vi "JEOL_SEM.vi"() -> ()   [LabVIEW 2016]
uses:
  cluster_fontsettings.ctl
  cluster_colorsettings.ctl
  cluster_spacing.ctl
  cluster_background.ctl
panel:
  out "picture":picture
  in  "save all images":bool
  in  "End Program":bool
  out "Resolution [px]":i16[](array[numeric])=[2560, 1920] caption="Picture resolution (X*Y = width x height) [pixel]"
  in  "Spacing":T1={"Background"={"use picture width"=FALSE, "Settings"={"add box below image"=FALSE, "extra width background"=30, "extra height background"=30, "x [px]"=50.0, "y [px]"=50.0}}, "Scalebar"={"height of bar [px]"=50.0, "width scaling factor"=1.0, "Precision"=0}}
  in  "Color settings":T3={"Background color"=0, "Information color"=16777215}
  in  "Font settings":T4={"Font"=0, "Font size [px]"=60, "Bold"=FALSE} {"Font" items=["Arial", "Arial Italic", "Arial Bold", "Arial Bold Italic", "Batang & BatangChe & Gungsuh & GungsuhChe", "Courier New", "Courier New Italic", "Courier New Bold", "Courier New Bold Italic", "DaunPenh", "DokChampa", "Estrangelo Edessa", "Euphemia", "Gautami", "Gautami Bold", "Vani", "Vani Bold", "Gulim & GulimChe & Dotum & DotumChe", "Impact", "Iskoola Pota", "Iskoola Pota Bold", "Kalinga", "Kalinga Bold", "Kartika", "Kartika Bold", "Khmer UI", "Khmer UI Bold", "Lao UI", "Lao UI Bold", "Latha", "Latha Bold", "Lucida Console", "Malgun Gothic", "Malgun Gothic Bold", "Mangal", "Mangal Bold", "Meiryo & Meiryo Italic & Meiryo UI & Meiryo UI Italic", "Meiryo Bold & Meiryo Bold Italic & Meiryo UI Bold & Meiryo UI Bold Italic", "Microsoft Himalaya", "Microsoft JhengHei", "Microsoft JhengHei Bold", "Microsoft YaHei", "Microsoft YaHei Bold", "MingLiU & PMingLiU & MingLiU_HKSCS", "MingLiU-ExtB & PMingLiU-ExtB & MingLiU_HKSCS-ExtB", "Mongolian Baiti", "MS Gothic & MS PGothic & MS UI Gothic", "MS Mincho & MS PMincho", "MV Boli", "Microsoft New Tai Lue", "Microsoft New Tai Lue Bold", "Nyala", "Microsoft PhagsPa", "Microsoft PhagsPa Bold", "Plantagenet Cherokee", "Raavi", "Raavi Bold", "Segoe Script", "Segoe Script Bold", "Segoe UI", "Segoe UI Bold", "Segoe UI Italic", "Segoe UI Bold Italic", "Segoe UI Semibold", "Segoe UI Light", "Segoe UI Symbol", "Shruti", "Shruti Bold", "SimSun & NSimSun", "SimSun-ExtB", "Sylfaen", "Microsoft Tai Le", "Microsoft Tai Le Bold", "Times New Roman", "Times New Roman Italic", "Times New Roman Bold", "Times New Roman Bold Italic", "Tunga", "Tunga Bold", "Vrinda", "Vrinda Bold", "Shonar Bangla", "Shonar Bangla Bold", "Microsoft Yi Baiti", "Tahoma", "Tahoma Bold", "Microsoft Sans Serif", "Angsana New", "Angsana New Italic", "Angsana New Bold", "Angsana New Bold Italic", "Aparajita", "Aparajita Bold", "Aparajita Bold Italic(TrueType)", "Aparajita Italic", "Cordia New", "Cordia New Italic", "Cordia New Bold", "Cordia New Bold Italic", "Ebrima", "Ebrima Bold", "Gisha", "Gisha Bold", "Kokila", "Kokila Bold", "Kokila Bold Italic(TrueType)", "Kokila Italic", "MoolBoran", "Symbol", "Utsaah", "Utsaah Bold", "Utsaah Bold Italic(TrueType)", "Utsaah Italic", "Vijaya", "Vijaya Bold", "Wingdings", "Modern", "Roman", "Script", "Andalus", "Arabic Typesetting", "Simplified Arabic", "Simplified Arabic Bold", "Simplified Arabic Fixed", "Sakkal Majalla", "Sakkal Majalla Bold", "Traditional Arabic", "Traditional Arabic Bold", "Aharoni Bold", "David", "David Bold", "FrankRuehl", "Levenim MT", "Levenim MT Bold", "Miriam", "Miriam Fixed", "Narkisim", "Rod", "FangSong", "SimHei", "KaiTi", "AngsanaUPC", "AngsanaUPC Italic", "AngsanaUPC Bold", "AngsanaUPC Bold Italic", "Browallia New", "Browallia New Italic", "Browallia New Bold", "Browallia New Bold Italic", "BrowalliaUPC", "BrowalliaUPC Italic", "BrowalliaUPC Bold", "BrowalliaUPC Bold Italic", "CordiaUPC", "CordiaUPC Bold", "CordiaUPC Bold Italic", "CordiaUPC Italic", "DilleniaUPC", "DilleniaUPC Italic", "DilleniaUPC Bold", "DilleniaUPC Bold Italic", "EucrosiaUPC", "EucrosiaUPC Italic", "EucrosiaUPC Bold", "EucrosiaUPC Bold Italic", "FreesiaUPC", "FreesiaUPC Italic", "FreesiaUPC Bold", "FreesiaUPC Bold Italic", "IrisUPC", "IrisUPC Italic", "IrisUPC Bold", "IrisUPC Bold Italic", "JasmineUPC", "JasmineUPC Italic", "JasmineUPC Bold", "JasmineUPC Bold Italic", "KodchiangUPC", "KodchiangUPC Italic", "KodchiangUPC Bold", "KodchiangUPC Bold Italic", "LilyUPC", "LilyUPC Italic", "LilyUPC Bold", "LilyUPC Bold Italic", "DFKai-SB", "Lucida Sans Unicode", "Arial Black", "Calibri", "Calibri Italic", "Calibri Bold", "Calibri Bold Italic", "Cambria & Cambria Math", "Cambria Italic", "Cambria Bold", "Cambria Bold Italic", "Candara", "Candara Italic", "Candara Bold", "Candara Bold Italic", "Comic Sans MS", "Comic Sans MS Bold", "Consolas", "Consolas Italic", "Consolas Bold", "Consolas Bold Italic", "Constantia", "Constantia Italic", "Constantia Bold", "Constantia Bold Italic", "Corbel", "Corbel Italic", "Corbel Bold", "Corbel Bold Italic", "Franklin Gothic Medium", "Franklin Gothic Medium Italic", "Gabriola", "Georgia", "Georgia Italic", "Georgia Bold", "Georgia Bold Italic", "Palatino Linotype", "Palatino Linotype Italic", "Palatino Linotype Bold", "Palatino Linotype Bold Italic", "Segoe Print", "Segoe Print Bold", "Trebuchet MS", "Trebuchet MS Italic", "Trebuchet MS Bold", "Trebuchet MS Bold Italic", "Verdana", "Verdana Italic", "Verdana Bold", "Verdana Bold Italic", "Webdings", "Courier 10,12,15", "MS Serif 8,10,12,14,18,24", "MS Sans Serif 8,10,12,14,18,24", "Small Fonts", "Small Fonts", "Arial Narrow", "Book Antiqua", "Bookman Old Style", "Century Gothic", "Garamond", "Monotype Corsiva", "Book Antiqua Bold", "Book Antiqua Bold Italic", "Book Antiqua Italic", "Arial Narrow Bold", "Arial Narrow Bold Italic", "Arial Narrow Italic", "Bookman Old Style Bold", "Bookman Old Style Bold Italic", "Bookman Old Style Italic", "Garamond Bold", "Garamond Italic", "Century Gothic Bold", "Century Gothic Bold Italic", "Century Gothic Italic", "DIN-Bold", "DIN-Regular", "DIN-Black", "BEYBNQ+InfoDispRegular-Roman", "motorhead Standard", "FENCES.TTF", "MTEXTRA.TTF", "Origin", "Roboto Condensed Light Italic", "Roboto Condensed Regular", "Roboto Condensed Bold Italic", "Roboto Condensed Italic", "Roboto Condensed Light", "LMSans10-Regular", "LMSans10-BoldOblique", "LMSans10-Oblique", "LMSans10-Bold", "LMSansDemiCond10-Oblique", "Roboto Condensed Bold", "FA123ALG", "FA123GRF", "Agency FB Fett", "Agency FB", "Algerian", "Arial Rounded MT Bold", "Baskerville Old Face", "Bauhaus 93", "Bell MT", "Bell MT Fett", "Bell MT Kursiv", "Bernard MT Condensed", "Bodoni MT Fett", "Bodoni MT Fett Kursiv", "Bodoni MT Black Kursiv", "Bodoni MT Black", "Bodoni MT Condensed Fett", "Bodoni MT Condensed Fett Kursiv", "Bodoni MT Condensed Kursiv", "Bodoni MT Condensed", "Bodoni MT Kursiv", "Bodoni MT Poster Compressed", "Bodoni MT", "Bradley Hand ITC", "Britannic Bold", "Berlin Sans FB Fett", "Berlin Sans FB Demi Fett", "Berlin Sans FB", "Broadway", "Brush Script MT Kursiv", "Bookshelf Symbol 7", "Californian FB Fett", "Californian FB Kursiv", "Californian FB", "Calisto MT", "Calisto MT Fett", "Calisto MT Fett Kursiv", "Calisto MT Kursiv", "Castellar", "Century Schoolbook", "Centaur", "Chiller", "Colonna MT", "Cooper Black", "Copperplate Gothic Bold", "Copperplate Gothic Light", "Curlz MT", "Elephant", "Elephant Kursiv", "Engravers MT", "Eras Bold ITC", "Eras Demi ITC", "Eras Light ITC", "Eras Medium ITC", "Felix Titling", "Forte", "Franklin Gothic Book", "Franklin Gothic Book Kursiv", "Franklin Gothic Demi", "Franklin Gothic Demi Cond", "Franklin Gothic Demi Kursiv", "Franklin Gothic Heavy", "Franklin Gothic Heavy Kursiv", "Franklin Gothic Medium Cond", "Freestyle Script", "French Script MT", "Footlight MT Light", "Gigi", "Gill Sans MT", "Gill Sans MT Fett", "Gill Sans MT Fett Kursiv", "Gill Sans MT Condensed", "Gill Sans MT Kursiv", "Gill Sans Ultra Bold Condensed", "Gill Sans Ultra Bold", "Gloucester MT Extra Condensed", "Gill Sans MT Ext Condensed Bold", "Goudy Old Style", "Goudy Old Style Fett", "Goudy Old Style Kursiv", "Goudy Stout", "Harlow Solid Italic", "Harrington", "Haettenschweiler", "High Tower Text", "High Tower Text Kursiv", "Imprint MT Shadow", "Informal Roman", "Blackadder ITC", "Edwardian Script ITC", "Kristen ITC", "Jokerman", "Juice ITC", "Kunstler Script", "Wide Latin", "Lucida Bright", "Lucida Bright Demibold", "Lucida Bright Demibold Italic", "Lucida Bright Italic", "Lucida Calligraphy Italic", "Lucida Fax", "Lucida Fax Halbfett", "Lucida Fax Halbfett Kursiv", "Lucida Fax Kursiv", "Lucida Handwriting Kursiv", "Lucida Sans", "Lucida Sans Halbfett", "Lucida Sans Halbfett Kursiv", "Lucida Sans Kursiv", "Lucida Sans Typewriter", "Lucida Sans Typewriter Fett", "Lucida Sans Typewriter Fett Schräg", "Lucida Sans Typewriter Schräg", "Magneto Fett", "Maiandra GD", "Matura MT Script Capitals", "Mistral", "Modern No. 20", "Niagara Engraved", "Niagara Solid", "OCR A Extended", "Old English Text MT", "Onyx", "MS Outlook", "Palace Script MT", "Papyrus", "Parchment", "Perpetua", "Perpetua Fett", "Perpetua Fett Kursiv", "Perpetua Kursiv", "Perpetua Titling MT Fett", "Perpetua Titling MT Mager", "Playbill", "Poor Richard", "Pristina", "Rage Italic", "Ravie", "MS Reference Sans Serif", "MS Reference Specialty", "Rockwell Condensed", "Rockwell Condensed Fett", "Rockwell", "Rockwell Fett", "Rockwell Fett Kursiv", "Rockwell Extra Bold", "Rockwell Kursiv", "Century Schoolbook Fett", "Century Schoolbook Fett Kursiv", "Century Schoolbook Kursiv", "Script MT Bold", "Showcard Gothic", "Snap ITC", "Stencil", "Tw Cen MT Fett", "Tw Cen MT Fett Kursiv", "Tw Cen MT Condensed Fett", "Tw Cen MT Condensed Extra Bold", "Tw Cen MT Condensed", "Tw Cen MT", "Tw Cen MT Kursiv", "Tempus Sans ITC", "Viner Hand ITC", "Vivaldi Kursiv", "Vladimir Script", "Digital Readout Upright", "Eurotherm Message Center", "Eurotherm Starburst", "Eurotherm Series 2000", "FreeSerif Fett-Kursiv", "FreeSerif Fett", "FreeSerif Mittel", "FreeSans Kursiv", "FreeSans Fett-Kursiv", "FreeSans Fett", "FreeSans Mittel", "FreeMono Kursiv", "FreeMono Fett-Kursiv", "FreeMono Fett", "FreeMono Standard", "FreeSerif Kursiv", "TeamViewer12", "Arial Unicode MS", "Century", "Gadugi", "Leelawadee", "Microsoft JhengHei & Microsoft JhengHei UI", "Microsoft Uighur", "Microsoft YaHei & Microsoft YaHei UI", "Segoe UI Semilight", "Wingdings 2", "Wingdings 3", "Gadugi Bold", "Leelawadee Bold", "Microsoft JhengHei Bold & Microsoft JhengHei UI Bold", "Microsoft Uighur Bold", "Microsoft YaHei Bold & Microsoft YaHei UI Bold", "Nirmala UI Bold", "Calibri Light Italic", "Nirmala UI", "Calibri Light", "Leipzig Fraktur Normal", "MT Extra"]}
  in  "save image":bool
  in  "Preview":bool
  in  "load image":bool
  in  "Path to directory to convert all files (only save image will work, so make sure settings are ok!)":path
  in  "Path to single file (png or txt with metadata)":path
  # "x and y are the distance between the\nlower left corner of the image and the\nlower left corner of the box"
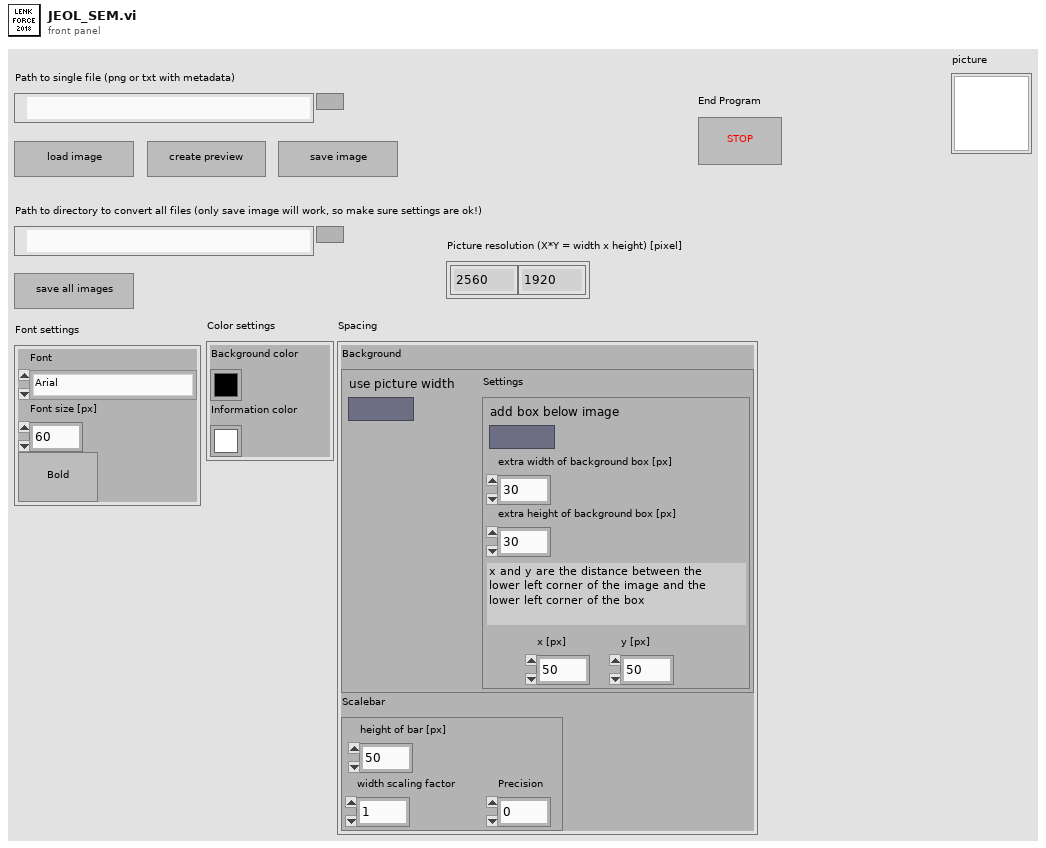
[diagram p1: front panel]
types:
  T1 = typedef "cluster_spacing.ctl" = cluster{"Background":T2, "Scalebar":cluster{"height of bar [px]":dbl, "width scaling factor":dbl, "Precision":i16}}
  T2 = typedef "cluster_background.ctl" = cluster{"use picture width":bool, "Settings":cluster{"add box below image":bool, "extra width background":i16, "extra height background":i16, "x [px]":dbl, "y [px]":dbl}}
  T3 = typedef "cluster_colorsettings.ctl" = cluster{"Background color":u32, "Information color":u32}
  T4 = typedef "cluster_fontsettings.ctl" = cluster{"Font":u16, "Font size [px]":i16, "Bold":bool}
  T5 = cluster{"Font Name:":string, "Size":i16, "Strikeout?":bool, "Italic?":bool, "Underline?":bool, "Outline?":bool, "Shadow?":bool, "Bold?":bool}
  T6 = typedef "cluster_metadata.ctl" = cluster{"FOV v":dbl, "FOV v unit":string, "FOV h":dbl, "FOV h unit":string, "Micron marker":dbl, "Micron marker unit":string, "Resolution h":i32, "Resolution v":i32, "Maginfication":i32}
  T7 = typedef "imagedata.ctl" = cluster{"image type":i32, "image depth":i32, "image":u8[], "mask":u8[], "colors":u32[], "Rectangle":cluster{"left":i16, "top":i16, "right":i16, "bottom":i16}}
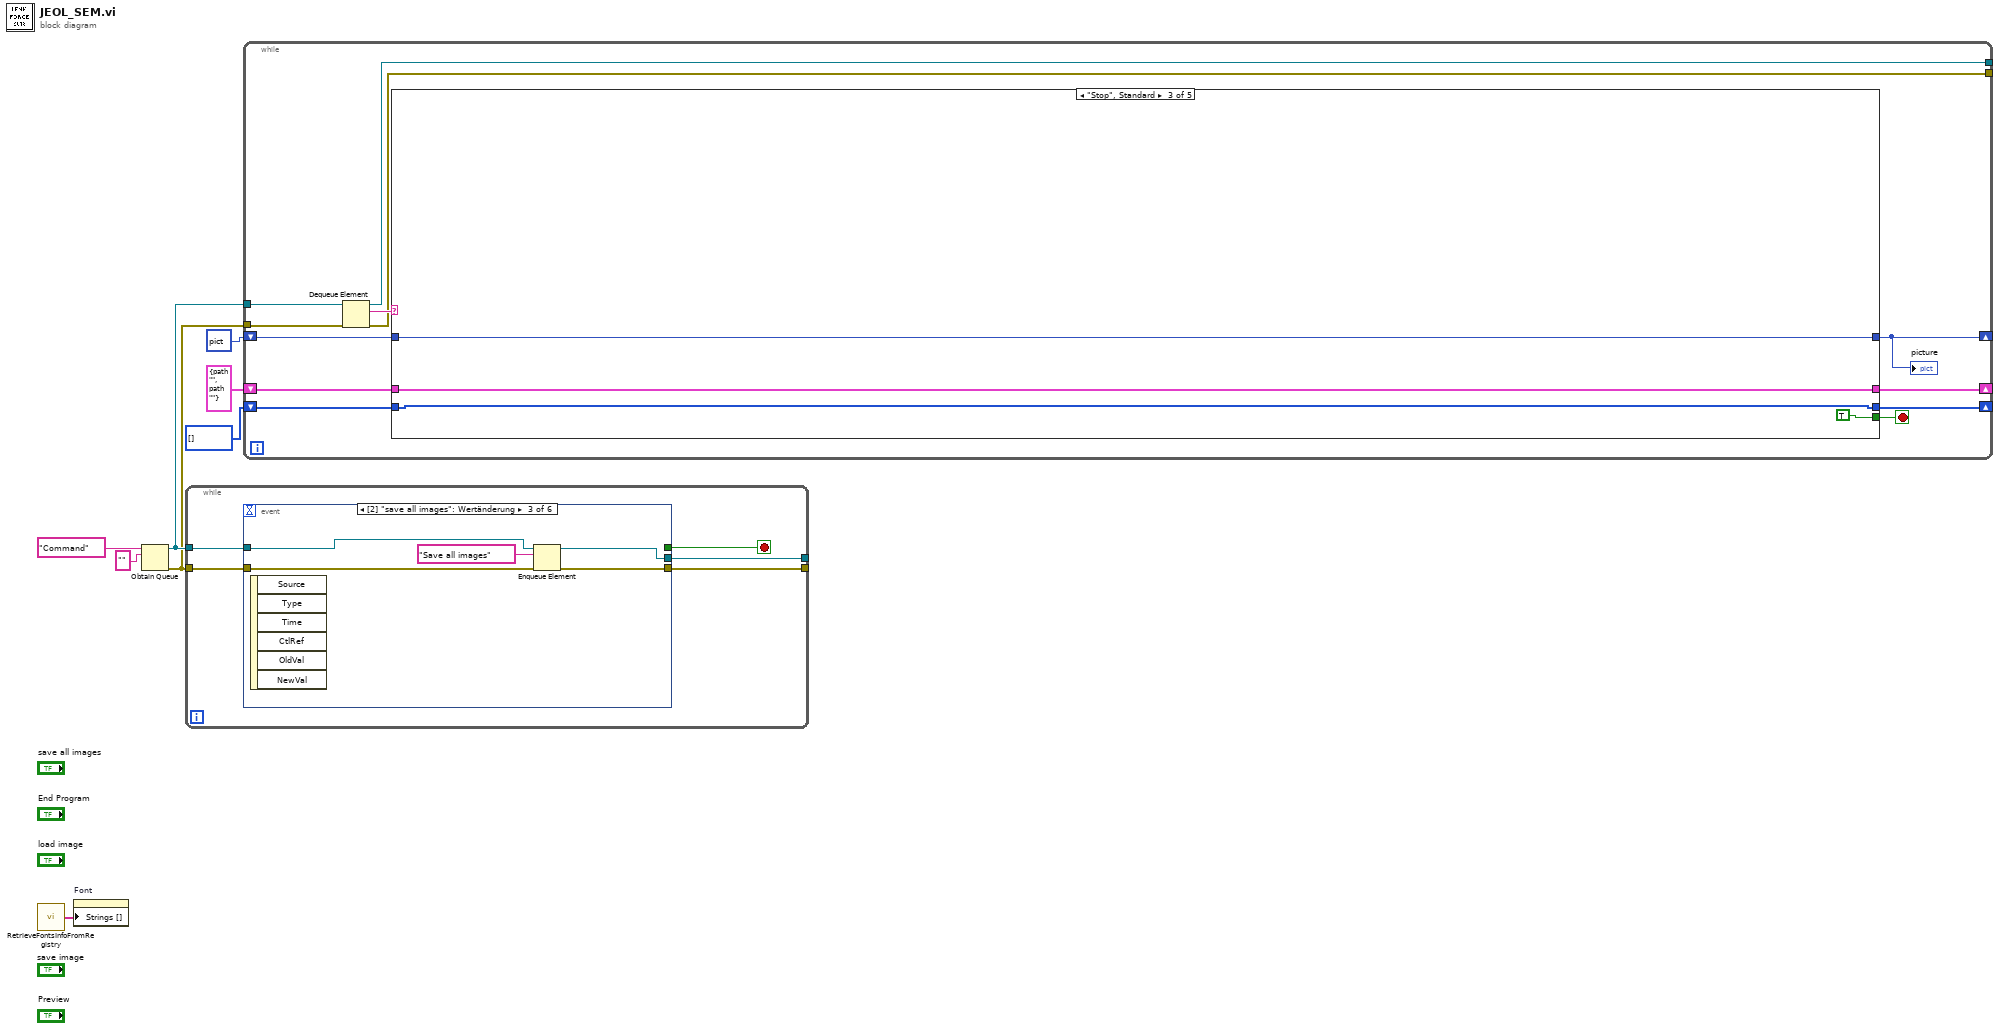
[diagram p0: block diagram]
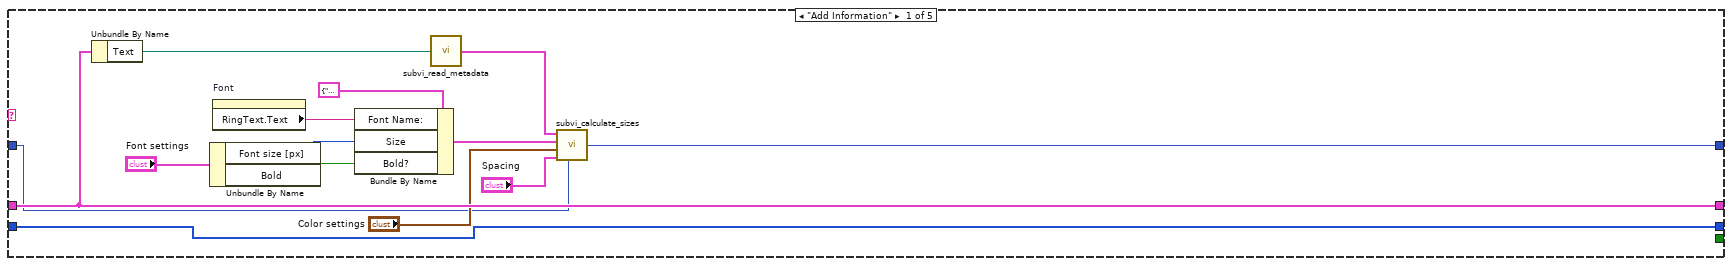
[diagram p2: hidden frame]
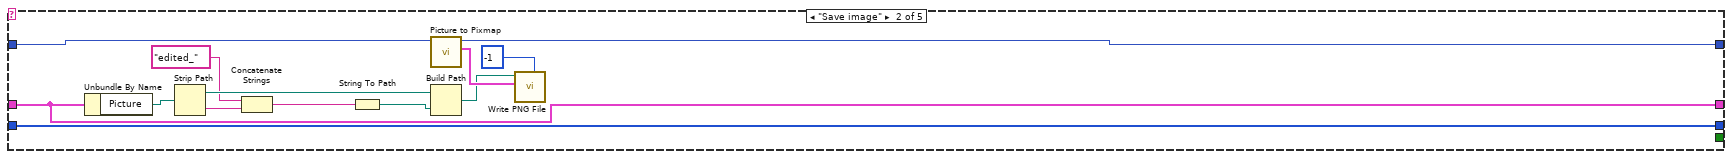
[diagram p3: hidden frame]
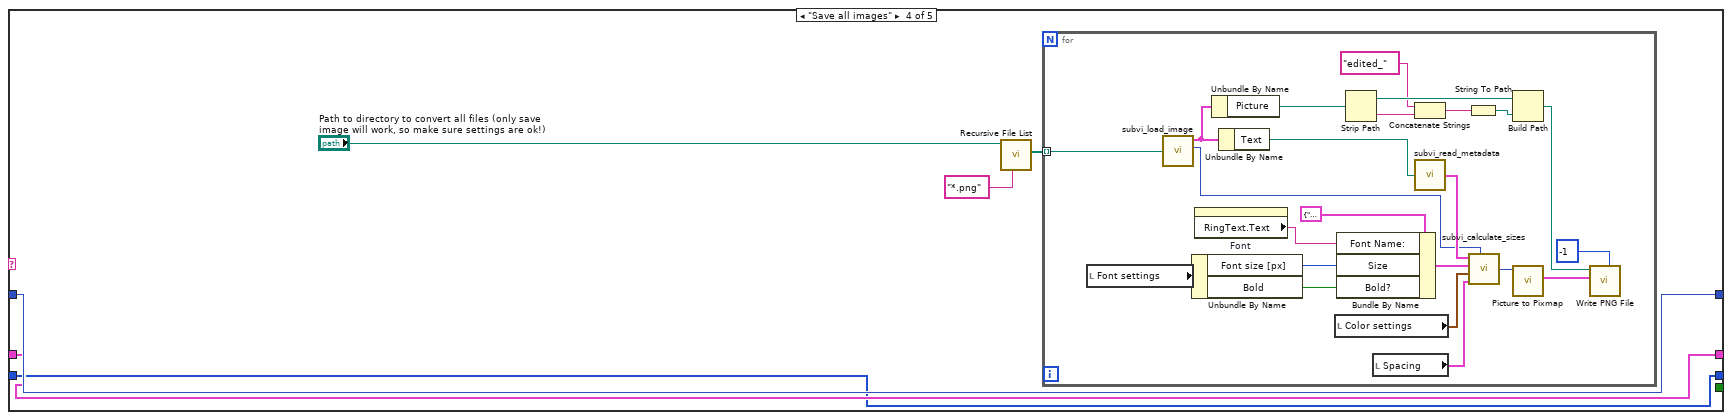
[diagram p4: hidden frame]
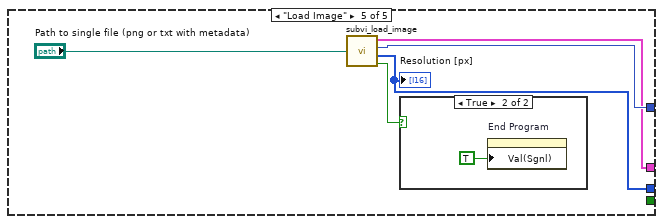
[diagram p5: hidden frame]
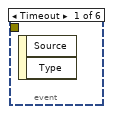
[diagram p7: hidden frame]
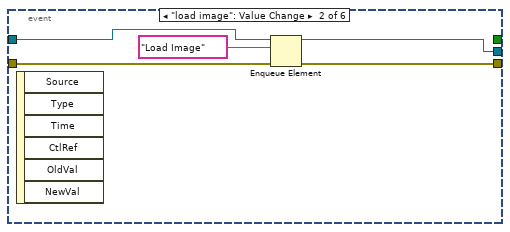
[diagram p8: hidden frame]
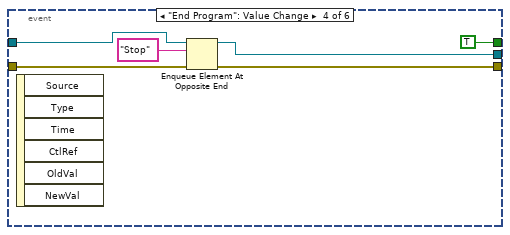
[diagram p9: hidden frame]
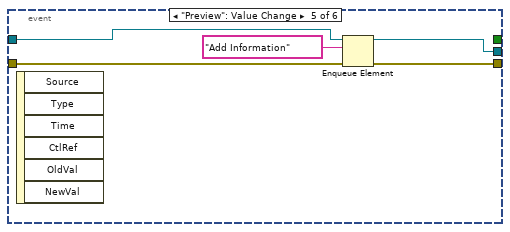
[diagram p10: hidden frame]
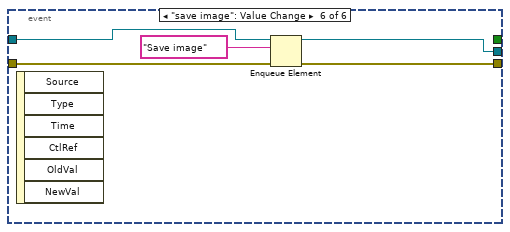
[diagram p11: hidden frame]
diagram:
  n1 = call "RetrieveFontsInfoFromRegistry.vi"() -> ("Fonts Installed"=w8:string[])
  n2 = property on="Font" class="Ring (strikt)"("Strings []"=w8) -> ()  [unwired: 2 in, 2 out]
  n3 = Obtain Queue(name (unnamed)="Command" ("Name (unbenannt)"), element data type="") -> (queue out=w6:refnum<queue>, error out=w4:errorcluster)  [unwired: 3 in, 1 out]
  n4 = while {
    tunnel: w6 -> [w13]
    tunnel: w4 -> [w12]
    tunnel: [w11] -> _
    tunnel: [w10] -> _
    stop <- w9 stop-if-true
    n5 = event shown="[2] \"save all images\": Wertänderung" {
      selector: _ -> [_ _ _ _ _ _]
      dyn-events: _ -> [_ _ _ _ _ _]
      timeout: _ -> [_ _ _ _ _ _]
      tunnel: w13 -> [_ w18 w22 w29 w34 w38]
      tunnel: w12 -> [_ w17 w21 w26 w33 w35]
      tunnel: [_ w15 w20 w28 w31 w37] -> w11
      tunnel: [_ w14 w19 w25 w32 w36] -> w10
      tunnel: [_ _ _ TRUE _ _] -> w9
      event Timeout {
        n6 = event-data() -> ()  [unwired: 1 in, 2 out]
      }
      event "load image": Value Change {
        n7 = event-data() -> ()  [unwired: 1 in, 6 out]
        n8 = Enqueue Element(queue=w18, element="Load Image" ("Element"), error in (no error)=w17) -> (queue out=w15:refnum<queue>, error out=w14:errorcluster)  [unwired: 1 in, 1 out]
      }
      event "save all images": Value Change {
        n9 = event-data() -> ()  [unwired: 1 in, 6 out]
        n10 = Enqueue Element(queue=w22, element="Save all images" ("Element"), error in (no error)=w21) -> (queue out=w20:refnum<queue>, error out=w19:errorcluster)  [unwired: 1 in, 1 out]
      }
      event "End Program": Value Change {
        n11 = event-data() -> ()  [unwired: 1 in, 6 out]
        n12 = Enqueue Element At Opposite End(queue=w29, element="Stop" ("Element"), error in (no error)=w26) -> (queue out=w28:refnum<queue>, error out=w25:errorcluster)  [unwired: 1 in, 1 out]
      }
      event "Preview": Value Change {
        n13 = event-data() -> ()  [unwired: 1 in, 6 out]
        n14 = Enqueue Element(queue=w34, element="Add Information" ("Element"), error in (no error)=w33) -> (queue out=w31:refnum<queue>, error out=w32:errorcluster)  [unwired: 1 in, 1 out]
      }
      event "save image": Value Change {
        n15 = event-data() -> ()  [unwired: 1 in, 6 out]
        n16 = Enqueue Element(queue=w38, element="Save image" ("Element"), error in (no error)=w35) -> (queue out=w37:refnum<queue>, error out=w36:errorcluster)  [unwired: 1 in, 1 out]
      }
    }
  }
  n17 = while {
    tunnel: w6 -> [w51]
    tunnel: w4 -> [w50]
    shift-right: [w48] -> _
    shift-left: picture data[5B] ("loaded picture") -> [w47]
    shift-right: [w46] -> _
    shift-left: i16[] [] ("Resolution [px]") -> [w45]
    shift-right: [w44] -> _
    shift-left: cluster{"Picture":path, "Text":path} {"Picture"=path "", "Text"=path ""} ("Paths to data") -> [w43]
    tunnel: [w41] -> _
    tunnel: [w40] -> _
    stop <- w42 stop-if-true
    n18 = Dequeue Element(queue=w51, error in (no error)=w50) -> (queue out=w41:refnum<queue>, element=w49:string, error out=w40:errorcluster)  [unwired: 1 in, 1 out]
    n19 = case shown="\"Stop\", Standard" w49 {
      tunnel: [w52 w75 w80 w85 w115] -> w48
      tunnel: w47 -> [w54 w76 w80 w85 _]
      tunnel: [w53 w69 w79 w83 w114] -> w46
      tunnel: w45 -> [w53 w69 w79 w83 _]
      tunnel: [w65 w70 w81 w84 w112] -> w44
      tunnel: w43 -> [w65 w70 w81 w84 _]
      tunnel: [_ _ TRUE _ _] -> w42
      frame "Add Information" {
        n20 = Unbundle By Name(w65) -> ("Text"=w64:path)
        n21 = Unbundle By Name("Font settings") -> ("Font size [px]"=w63:i16, "Bold"=w62:bool)
        n22 = property on="Font" class="Ring (strikt)"() -> ("RingText.Text"=w59:string)  [unwired: 2 in, 2 out]
        n23 = Bundle By Name(cluster=T5 {"Font Name:"="Arial", "Size"=12, "Strikeout?"=FALSE, "Italic?"=FALSE, "Underline?"=FALSE, "Outline?"=FALSE, "Shadow?"=FALSE, "Bold?"=FALSE} ("[user-specified font]"), "Font Name:"=w59, "Size"=w63, "Bold?"=w62) -> (w57:T5)
        n24 = call "subvi_read_metadata.vi"("Pfad"=w64) -> ("Metadata"=w58:T6)
        n25 = call "subvi_calculate_sizes.vi"("Metadata"=w58, "font settings"=w57, "Color settings"="Color settings", "Spacing"="Spacing", "loaded picture"=w54) -> ("modified pictures"=w52:picture)
      }
      frame "Save image" {
        n26 = Unbundle By Name(w70) -> ("Picture"=w74:path)
        n27 = Strip Path(path=w74) -> (stripped path=w73:path, name=w68:string)
        n28 = Concatenate Strings("edited_" ("String"), w68) -> (w66:string)
        n29 = String To Path(string=w66) -> (path=w72:path)
        n30 = call <vilib>:"Picture to Pixmap.vi"("picture"=w76) -> ("image data"=w77:T7, "new picture"=w75:picture)  [unwired: 9 in]
        n31 = Build Path(base path=w73, name or relative path=w72) -> (appended path=w71:path)
        n32 = call <vilib>:"Write PNG File.vi"("compression (default)"=-1, "image data"=w77, "path to PNG file"=w71) -> ()  [unwired: 7 in, 2 out]
      }
      frame "Stop", Default {
      }
      frame "Save all images" {
        n33 = call <vilib>:"Recursive File List.vi"("pattern"="*.png", "Folder Path"="Path to directory to convert all files (only save image will work, so make sure settings are ok!)") -> ("All Files in Dir"=w86:path[])  [unwired: 5 in, 4 out]
        n34 = for {
          tunnel: w86 -> [w111] mode=indexing
          n35 = local read "Font settings"() -> (w102:T4)
          n36 = call "subvi_load_image.vi"("Path to single file (png or txt with metadata)"=w111) -> ("Paths to data"=w90:cluster{"Picture":path, "Text":path}, "loaded picture"=w104:picture)  [unwired: 2 out]
          n37 = Unbundle By Name(w102) -> ("Font size [px]"=w110:i16, "Bold"=w109:bool)
          n38 = property on="Font" class="Ring (strikt)"() -> ("RingText.Text"=w107:string)  [unwired: 2 in, 2 out]
          n39 = Unbundle By Name(w90) -> ("Picture"=w97:path)
          n40 = Unbundle By Name(w90) -> ("Text"=w103:path)
          n41 = local read "Color settings"() -> (w101:T3)
          n42 = Bundle By Name(cluster=T5 {"Font Name:"="Arial", "Size"=12, "Strikeout?"=FALSE, "Italic?"=FALSE, "Underline?"=FALSE, "Outline?"=FALSE, "Shadow?"=FALSE, "Bold?"=FALSE} ("[user-specified font]"), "Font Name:"=w107, "Size"=w110, "Bold?"=w109) -> (w105:T5)
          n43 = Strip Path(path=w97) -> (stripped path=w96:path, name=w93:string)
          n44 = local read "Spacing"() -> (w100:T1)
          n45 = Concatenate Strings("edited_" ("String"), w93) -> (w91:string)
          n46 = call "subvi_read_metadata.vi"("Pfad"=w103) -> ("Metadata"=w106:T6)
          n47 = String To Path(string=w91) -> (path=w95:path)
          n48 = call "subvi_calculate_sizes.vi"("Metadata"=w106, "font settings"=w105, "Color settings"=w101, "Spacing"=w100, "loaded picture"=w104) -> ("modified pictures"=w89:picture)
          n49 = Build Path(base path=w96, name or relative path=w95) -> (appended path=w94:path)
          n50 = call <vilib>:"Picture to Pixmap.vi"("picture"=w89) -> ("image data"=w98:T7)  [unwired: 9 in, 1 out]
          n51 = call <vilib>:"Write PNG File.vi"("compression (default)"=-1, "image data"=w98, "path to PNG file"=w94) -> ()  [unwired: 7 in, 2 out]
        }
      }
      frame "Load Image" {
        n52 = call "subvi_load_image.vi"("Path to single file (png or txt with metadata)"="Path to single file (png or txt with metadata)") -> ("Paths to data"=w112:cluster{"Picture":path, "Text":path}, "loaded picture"=w115:picture, "Resolution [px]"=w114:i16[], "Stop"=w113:bool)
        "Resolution [px]" <- w114
        n53 = case shown="True" w113 {
          frame False {
          }
          frame True {
            n54 = property on="End Program" class="Bool."("Val(Sgnl)"=TRUE ("Wert (signalisierend)")) -> ()  [unwired: 2 in, 2 out]
          }
        }
      }
    }
    "picture" <- w48
  }
